vi "MissionLocation.vi"(8 "Error In":errorcluster, 11 "Idle in":refnum<class "Idle.lvclass">) -> (0 "Error Out":errorcluster, 2 "element":T1 {"North" format="%#_10f"; "East" format="%#_8f"}, 3 "Idle out":refnum<class "Idle.lvclass">)   [LabVIEW 2013, in "Idle.lvclass"]
doc: "The general location of the mission for maps and such. In this case, it's the point to get to - the robot's current location, fed in at creation time."
uses:
  Idle.lvclass
  Data/TypeDefs/UTM Location.ctl
  GenericMission/GenericMission.lvclass
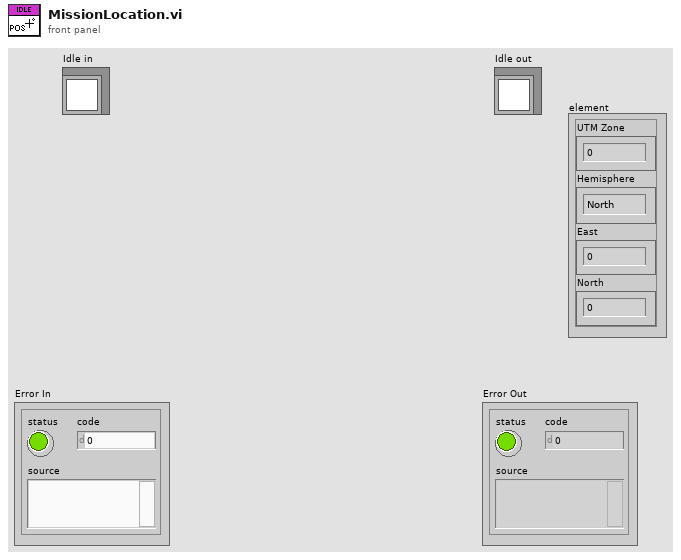
[diagram p1: front panel]
types:
  T1 = typedef "UTM Location.ctl" = cluster{"UTM Zone":dbl, "Hemisphere":enum16{"North", "South"}, "East":dbl, "North":dbl}
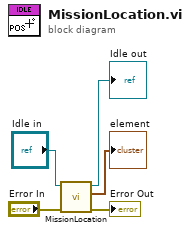
[diagram p0: block diagram]
diagram:
  n1 = call-parent "MissionLocation.vi"("Error In"="Error In", "GenericMission in"="Idle in") -> ("Error Out"=→"Error Out":errorcluster, "element"=→"element":T1, "GenericMission out"=→"Idle out":refnum<class "Idle.lvclass">)  [unwired: 7 in]
